vi "close hardware.vi"(8 "Error in":errorcluster) -> (0 "error out":errorcluster)   [LabVIEW 2020]
uses:
  <vilib>/ActorFramework/Stop Msg/Stop Msg.lvclass
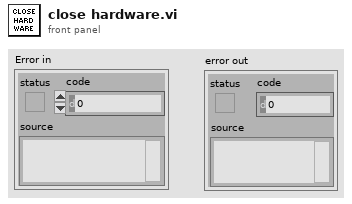
[diagram p1: front panel]
types:
  T1 = typedef "EquipmentCluster.ctl" = cluster{"Device":string, "Function":string, "Name":string, "Driver":string, "Address":string, "Device_queue":refnum<class "Message Enqueuer.lvclass">}
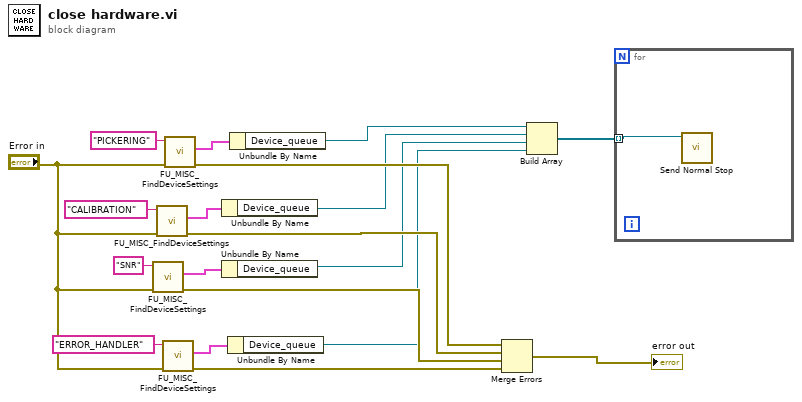
[diagram p0: block diagram]
diagram:
  n1 = call "FU_MISC_FindDeviceSettings.vi"("ErrorIn"="Error in", "DeviceID"="SNR") -> ("ErrorOut"=w8:errorcluster, "Settings"=w14:T1)  [unwired: 7 in, 1 out]
  n2 = call "FU_MISC_FindDeviceSettings.vi"("ErrorIn"="Error in", "DeviceID"="CALIBRATION") -> ("ErrorOut"=w7:errorcluster, "Settings"=w17:T1)  [unwired: 7 in, 1 out]
  n3 = call "FU_MISC_FindDeviceSettings.vi"("ErrorIn"="Error in", "DeviceID"="ERROR_HANDLER") -> ("ErrorOut"=w9:errorcluster, "Settings"=w12:T1)  [unwired: 7 in, 1 out]
  n4 = call "FU_MISC_FindDeviceSettings.vi"("ErrorIn"="Error in", "DeviceID"="PICKERING") -> ("ErrorOut"=w6:errorcluster, "Settings"=w18:T1)  [unwired: 7 in, 1 out]
  n5 = Unbundle By Name(w17) -> ("Device_queue"=w4:refnum<class "Message Enqueuer.lvclass">)
  n6 = Unbundle By Name(w14) -> ("Device_queue"=w3:refnum<class "Message Enqueuer.lvclass">)
  n7 = Unbundle By Name(w12) -> ("Device_queue"=w2:refnum<class "Message Enqueuer.lvclass">)
  n8 = Unbundle By Name(w18) -> ("Device_queue"=w5:refnum<class "Message Enqueuer.lvclass">)
  n9 = Merge Errors(w6, w7, w8, w9) -> (→"error out":errorcluster)
  n10 = Build Array(w5, w4, w3, w2) -> (w1:refnum<class "Message Enqueuer.lvclass">[])
  n11 = for {
    tunnel: w1 -> [w20] mode=indexing
    n12 = call <vilib>:"Send Normal Stop.vi"("Message Enqueuer"=w20) -> ()  [unwired: 10 in, 1 out]
  }
